vi "Oracle to Array.vi"(8 "error in":errorcluster, 11 "string in":string) -> (0 "error out":errorcluster, 1 "Empty?":bool, 3 "list out":T1[](array[typedef]) {"Last Updated" format="%<%x>T"})   [LabVIEW 2018]
uses:
  SR Cluster.ctl
  SR Status.ctl
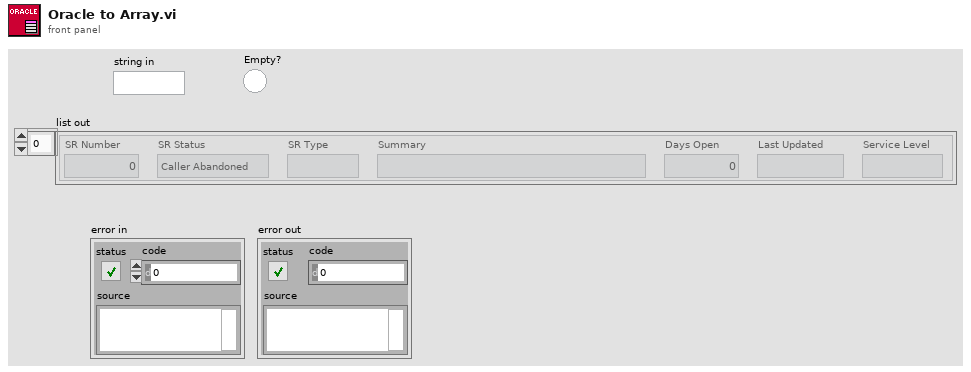
[diagram p1: front panel]
types:
  T1 = typedef "SR Cluster.ctl" = cluster{"SR Number":i32, "SR Type":string, "Summary":string, "Days Open":dbl, "Last Updated":timestamp, "Service Level":string, "SR Status":T2}
  T2 = typedef "SR Status.ctl" = enum16{"Caller Abandoned", "Created in Error", "Expired", "Forum Resolved AE", "Forum Resolved Customer", "IN WORK", "IN WORK Collab with AES", "IN WORK Collab with PSE", "IN WORK Collab with SE", "IN WORK Customer Added Note", "IN WORK Escalation", "IN WORK Wait on Customer", "Open", "Potentially Resolved", "Presumed Resolved", "RMA Approved for Return", "Resolved"}
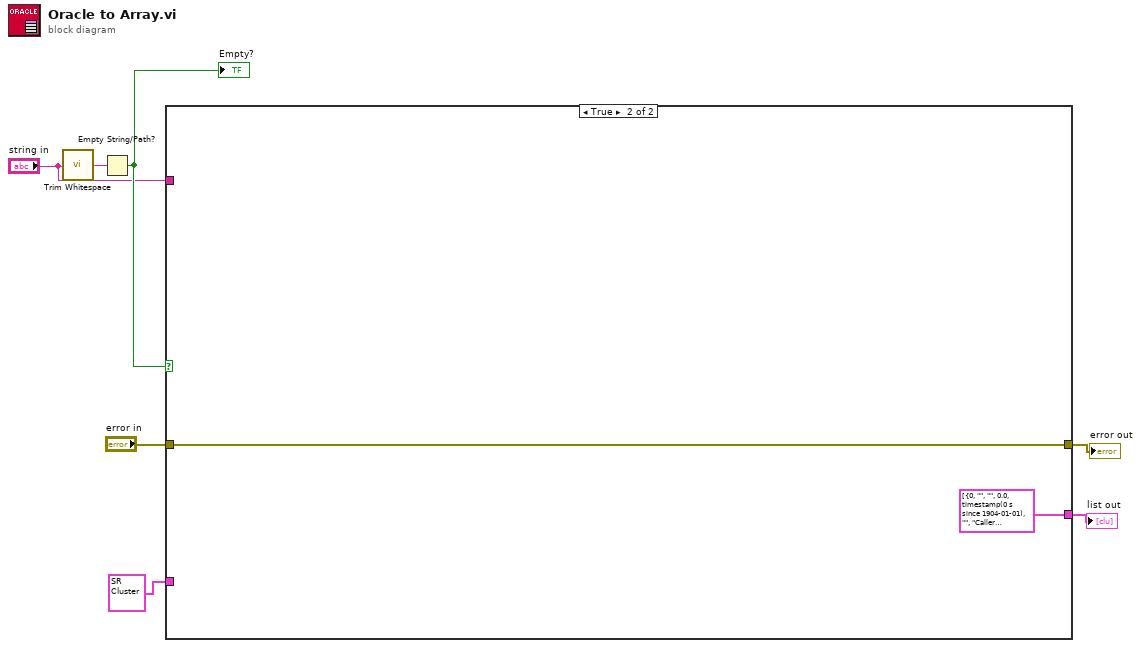
[diagram p0: block diagram]
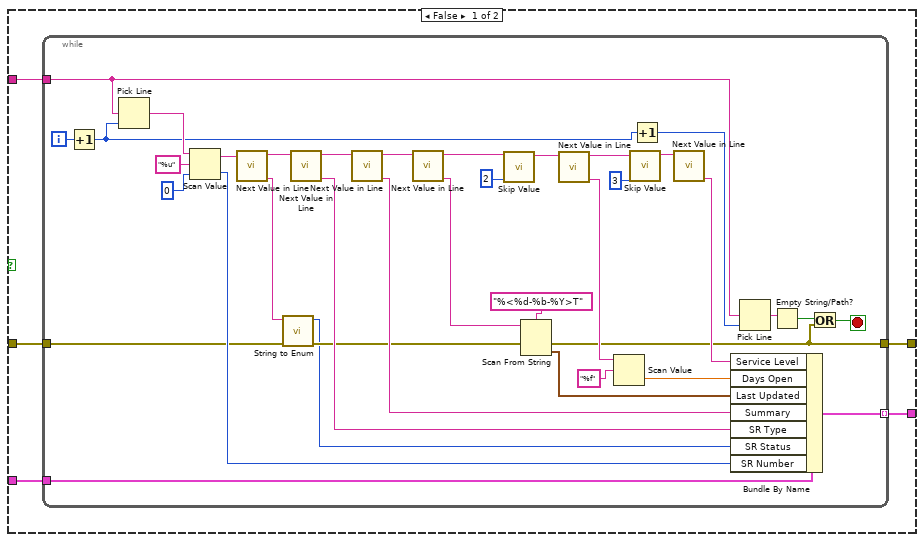
[diagram p2: hidden frame]
diagram:
  n1 = call <vilib>:"Trim Whitespace.vi"("string"="string in") -> ("trimmed string"=w5:string)  [unwired: 1 in]
  n2 = Empty String/Path?(string/path=w5) -> (empty?=w4:bool)
  "Empty?" <- w4
  n3 = case shown="True" w4 {
    tunnel: [w12 T1[] [{"SR Number"=0, "SR Type"="", "Summary"="", "Days Open"=0.0, "Last Updated"=timestamp(0 s since 1904-01-01), "Service Level"="", "SR Status"=enum."Caller Abandoned"}]] -> w7
    tunnel: [w11 w51] -> w6
    tunnel: "string in" -> [w10 _]
    tunnel: "error in" -> [w9 w51]
    tunnel: T1 {"SR Number"=0, "SR Type"="", "Summary"="", "Days Open"=0.0, "Last Updated"=timestamp(0 s since 1904-01-01), "Service Level"="", "SR Status"=enum."Caller Abandoned"} ("SR Cluster") -> [w8 _]
    frame False {
      n4 = while {
        tunnel: [w36] -> w12 mode=indexing
        tunnel: [w17] -> w11
        tunnel: w9 -> [w15]
        tunnel: w10 -> [w23]
        tunnel: w8 -> [w22]
        i -> [w21]
        stop <- w19 stop-if-true
        n5 = Increment(x=w21) -> (x+1=w20:i32)
        n6 = Pick Line(multi-line string=w23, line index=w20) -> (output string=w49:string)  [unwired: 1 in]
        n7 = Scan Value(string=w49, format string="%u", default (0 dbl)=0) -> (output string=w46:string, value=w42:i32)
        n8 = call "Next Value in Line.vi"("string in"=w46) -> ("value"=w16:string, "rest of string"=w45:string)  [unwired: 9 in]
        n9 = call "String to Enum.vi"("error in"=w15, "string in"=w16) -> ("error out"=w14:errorcluster, "enum out"=w13:T2)  [unwired: 8 in]
        n10 = call "Next Value in Line.vi"("string in"=w45) -> ("value"=w41:string, "rest of string"=w44:string)  [unwired: 9 in]
        n11 = call "Next Value in Line.vi"("string in"=w44) -> ("value"=w40:string, "rest of string"=w43:string)  [unwired: 9 in]
        n12 = call "Next Value in Line.vi"("string in"=w43) -> ("value"=w28:string, "rest of string"=w27:string)  [unwired: 9 in]
        n13 = call "Skip Value.vi"("How Many?"=2, "string in"=w27) -> ("string out"=w29:string)  [unwired: 9 in]
        n14 = Scan From String(format string="%<%d-%b-%Y>T", input string=w28, error in=w14) -> (error out=w17:errorcluster, output 1=w32:timestamp)  [unwired: 2 in, 2 out]
        n15 = call "Next Value in Line.vi"("string in"=w29) -> ("value"=w26:string, "rest of string"=w30:string)  [unwired: 9 in]
        n16 = Scan Value(string=w26, format string="%f") -> (value=w33:dbl)  [unwired: 1 in, 1 out]
        n17 = call "Skip Value.vi"("How Many?"=3, "string in"=w30) -> ("string out"=w31:string)  [unwired: 9 in]
        n18 = Increment(x=w20) -> (x+1=w34:i32)
        n19 = call "Next Value in Line.vi"("string in"=w31) -> ("value"=w37:string)  [unwired: 9 in, 1 out]
        n20 = Bundle By Name(cluster=w22, "Service Level"=w37, "Days Open"=w33, "Last Updated"=w32, "Summary"=w40, "SR Type"=w41, "SR Status"=w13, "SR Number"=w42) -> (w36:T1)
        n21 = Pick Line(multi-line string=w23, line index=w34) -> (output string=w35:string)  [unwired: 1 in]
        n22 = Empty String/Path?(string/path=w35) -> (empty?=w18:bool)
        n23 = Or(x=w18, y=w17) -> (x .or. y?=w19:bool)
      }
    }
    frame True {
    }
  }
  "list out" <- w7
  "error out" <- w6
